vi "Scripting_Project show item in tree.vi"() -> ()   [LabVIEW 2026]
panel:
  out "Item ID":string
  out "Selected Item":string
  out "Current Name":string
  in  "COPY":bool
  in  "stop":bool
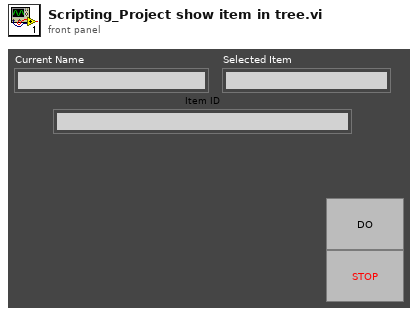
[diagram p1: front panel]
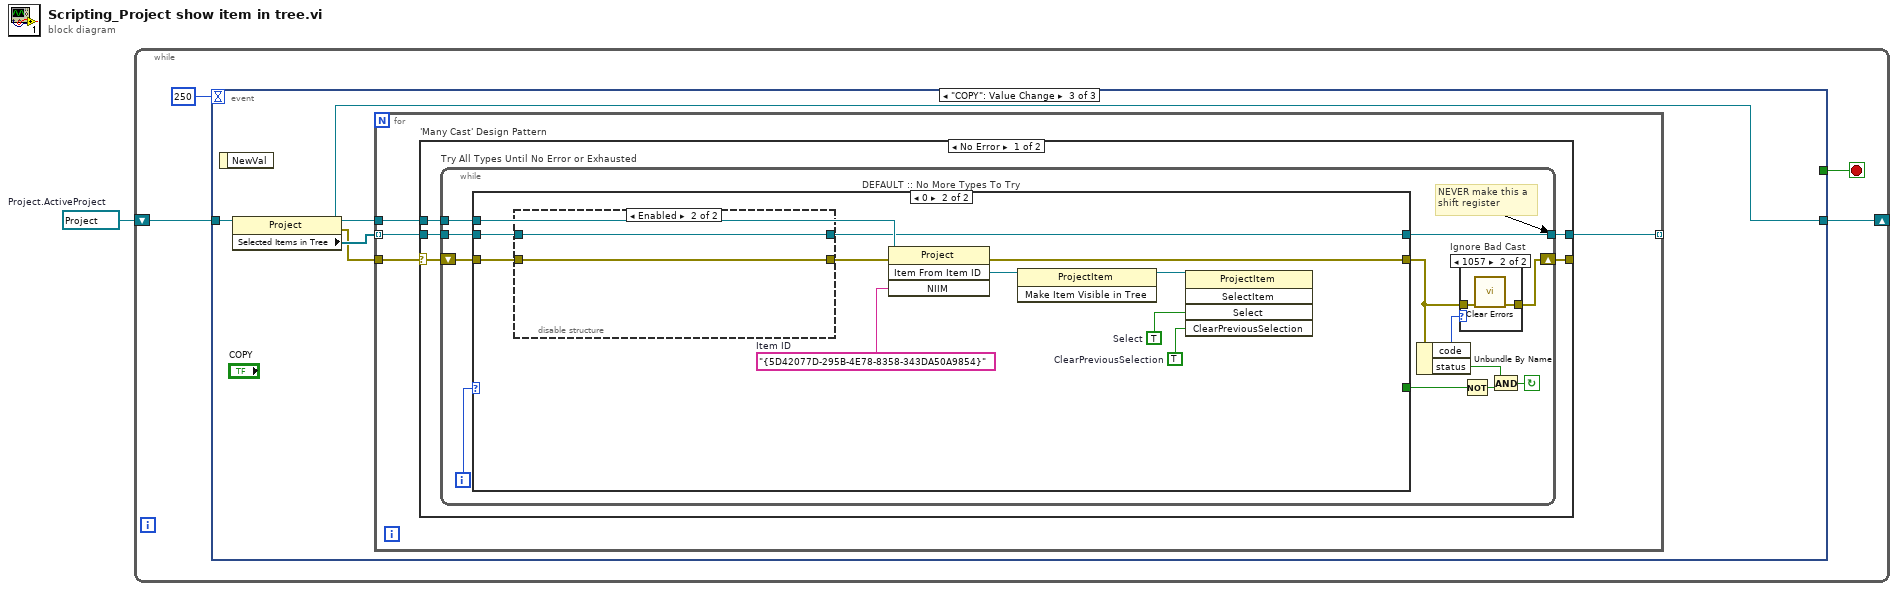
[diagram p0: block diagram]
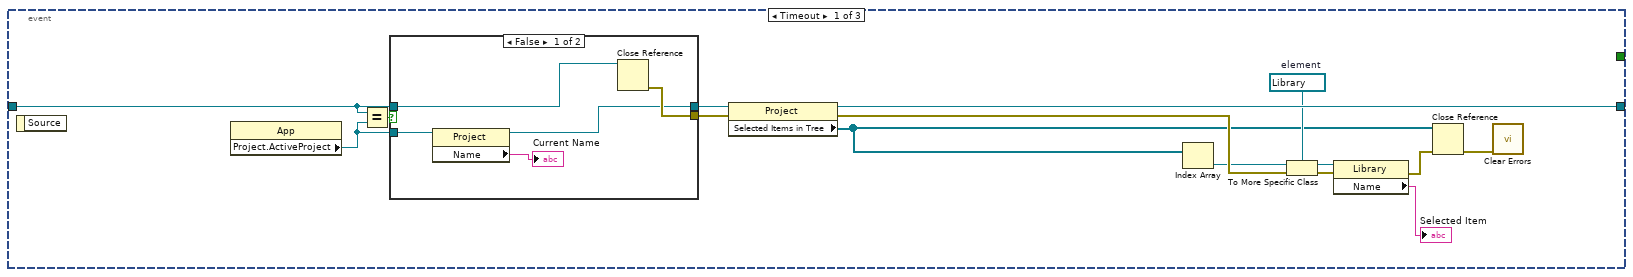
[diagram p2: hidden frame]
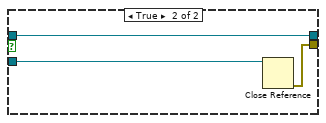
[diagram p3: hidden frame]
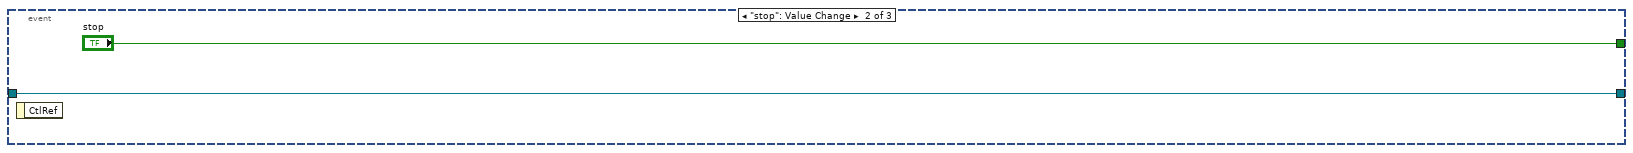
[diagram p4: hidden frame]
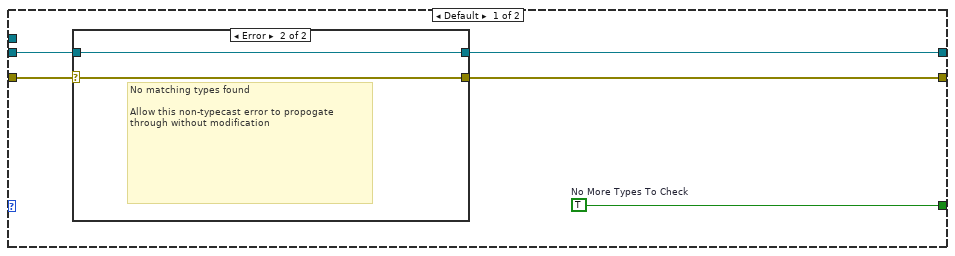
[diagram p6: hidden frame]
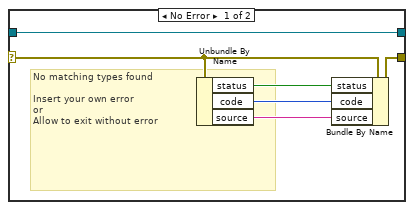
[diagram p7: hidden frame]
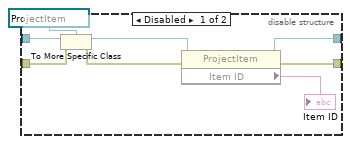
[diagram p8: hidden frame]
diagram:
  w1 = refnum<vi> refnum  # Project.ActiveProject
  n1 = while {
    shift-right: [w5] -> _
    shift-left: w1 -> [w4]
    stop <- w3 stop-if-true
    n2 = event shown="[2] \"COPY\": Value Change" {
      selector: _ -> [_ _ _]
      dyn-events: _ -> [_ _ _]
      timeout: 250 -> [_ _ _]
      tunnel: [w14 w30 w31] -> w5
      tunnel: w4 -> [w17 w30 w34]
      tunnel: [_ "stop" _] -> w3
      event Timeout {
        w8 = refnum<vi> refnum  # element
        n3 = event-data() -> ()  [unwired: 1 in, 1 out]
        n4 = property class="App"() -> ("Project.ActiveProject"=w18:refnum<vi>)  [unwired: 2 in, 2 out]
        n5 = Equal?(x=w17, y=w18) -> (x = y?=w19:bool)
        n6 = case shown="False" w19 {
          tunnel: w18 -> [w23 w28]
          tunnel: w17 -> [w25 w27]
          tunnel: [w22 w27] -> w15
          tunnel: [w24 w26] -> w11
          frame False {
            n7 = property class="Project"(reference=w23) -> (reference out=w22:refnum<vi>, "Name"=→"Current Name":string)  [unwired: 1 in, 1 out]
            n8 = Close Reference(reference=w25) -> (error out=w24:errorcluster)  [unwired: 1 in]
          }
          frame True {
            n9 = Close Reference(reference=w28) -> (error out=w26:errorcluster)  [unwired: 1 in]
          }
        }
        n10 = property class="Project"(reference=w15, error in=w11) -> (reference out=w14:refnum<vi>, error out=w20:errorcluster, "Selected Items in Tree"=w7:refnum<vi>[])
        n11 = Index Array(array=w7) -> (element=w13:refnum<vi>)  [unwired: 1 in]
        n12 = To More Specific Class(target class=w8, reference=w13, error in=w20) -> (specific class reference=w12:refnum<vi>, error out=w10:errorcluster)
        n13 = property class="Library"(reference=w12, error in=w10) -> (error out=w16:errorcluster, "Name"=→"Selected Item":string)  [unwired: 1 out]
        n14 = Close Reference(reference=w7, error in (no error)=w16) -> (error out=w9:errorcluster)
        n15 = call <vilib>:"Clear Errors.vi"("error in (no error)"=w9) -> ()  [unwired: 5 in, 2 out]
      }
      event "stop": Value Change {
        n16 = event-data() -> ()  [unwired: 1 in, 1 out]
      }
      event "COPY": Value Change {
        n17 = event-data() -> ()  [unwired: 1 in, 1 out]
        n18 = property class="Project"(reference=w34) -> (reference out=w31:refnum<vi>, error out=w32:errorcluster, "Selected Items in Tree"=w33:refnum<vi>[])  [unwired: 1 in]
        n19 = for {
          tunnel: w33 -> [w38] mode=indexing
          tunnel: w32 -> [w37]
          tunnel: [w36] -> _ mode=indexing
          tunnel: w31 -> [w35]
          n20 = case "'Many Cast' Design Pattern" shown="No Error" w37 {
            selector: w37 -> [w40 w94]
            tunnel: w38 -> [w43 w93]
            tunnel: [w42 w93] -> w36
            tunnel: [w41 w94] -> _
            tunnel: w35 -> [w39 _]
            frame No Error {
              n21 = while "Try All Types Until No Error or Exhausted" {
                tunnel: w43 -> [w55]
                tunnel: [w54] -> w42
                shift-right: [w47] -> w41
                shift-left: w40 -> [w49]
                tunnel: w39 -> [w44]
                i -> [w53]
                stop <- w52 continue-if-true
                # "NEVER make this a\nshift register"
                n22 = case "DEFAULT :: No More Types To Try" shown="0" w53 {
                  tunnel: w49 -> [w60 w82]
                  tunnel: w55 -> [w61 w81]
                  tunnel: [w62 w75] -> w54
                  tunnel: [w59 w79] -> w46
                  tunnel: [w63 _] -> w51
                  tunnel: w44 -> [_ w77]
                  frame Default {
                    w63 = TRUE  # No More Types To Check
                    n23 = case shown="Error" w60 {
                      selector: w60 -> [w67 w70]
                      tunnel: [w69 w71] -> w62
                      tunnel: w61 -> [w69 w71]
                      tunnel: [w68 w70] -> w59
                      frame No Error {
                        # "No matching types found\n\nInsert your own error \nor\nAllow to exit without error"
                        n24 = Unbundle By Name(w67) -> ("status"=w66:bool, "code"=w65:i32, "source"=w64:string)
                        n25 = Bundle By Name(cluster=w67, "status"=w66, "code"=w65, "source"=w64) -> (w68:errorcluster)
                      }
                      frame Error {
                        # "No matching types found\n\nAllow this non-typecast error to propogate through without modification"
                      }
                    }
                  }
                  frame 0 {
                    w72 = TRUE  # ClearPreviousSelection
                    w73 = TRUE  # Select
                    w78 = "{5D42077D-295B-4E78-8358-343DA50A9854}"  # Item ID
                    n26 = disable-structure shown="Enabled" {
                      disable-tunnel: w82 -> [w90 w92]
                      disable-tunnel: w81 -> [w88 w91]
                      disable-tunnel: [w85 w92] -> w80
                      disable-tunnel: [w84 w91] -> w75
                      frame Disabled {
                        n27 = To More Specific Class(target class=refnum<vi> refnum ("Waveform Chart"), reference=w88, error in=w90) -> (specific class reference=w86:refnum<vi>, error out=w87:errorcluster)
                        n28 = property class="ProjectItem"(reference=w86, error in=w87) -> (reference out=w84:refnum<vi>, error out=w85:errorcluster, "Item ID"=→"Item ID":string)
                      }
                      frame Enabled {
                      }
                    }
                    n29 = invoke class="Project" method="Item From Item ID"(reference=w77, error in=w80, "NIIM"=w78) -> (error out=w79:errorcluster, "GetItemFromNIIM"=w76:refnum<vi>)  [unwired: 1 in, 2 out]
                    n30 = invoke class="ProjectItem" method="Make Item Visible in Tree"(reference=w76) -> (reference out=w74:refnum<vi>)  [unwired: 2 in, 2 out]
                    n31 = invoke class="ProjectItem" method="SelectItem"(reference=w74, "Select"=w73, "ClearPreviousSelection"=w72) -> ()  [unwired: 2 in, 5 out]
                  }
                }
                n32 = Unbundle By Name(w46) -> ("code"=w45:i32, "status"=w48:bool)
                n33 = case "Ignore Bad Cast" shown="1057" w45 {
                  tunnel: [w56 w58] -> w47
                  tunnel: w46 -> [w56 w57]
                  frame Default {
                  }
                  frame 1057 {
                    n34 = call <vilib>:"Clear Errors.vi"("error in (no error)"=w57) -> ("error out"=w58:errorcluster)  [unwired: 5 in, 1 out]
                  }
                }
                n35 = Not(x=w51) -> (.not. x?=w50:bool)
                n36 = And(x=w48, y=w50) -> (x .and. y?=w52:bool)
              }
            }
            frame Error {
            }
          }
        }
      }
    }
  }
